vi "MatchInterface.vi"(8 "error in (no error)":errorcluster, 10 "Interface 2":T1, 11 "Interface 1":T1) -> (0 "error out":errorcluster, 2 "Wildcard":bool, 3 "Matches":bool)   [LabVIEW 2017]
uses:
  <vilib>/WebServerConfig/Interface.ctl
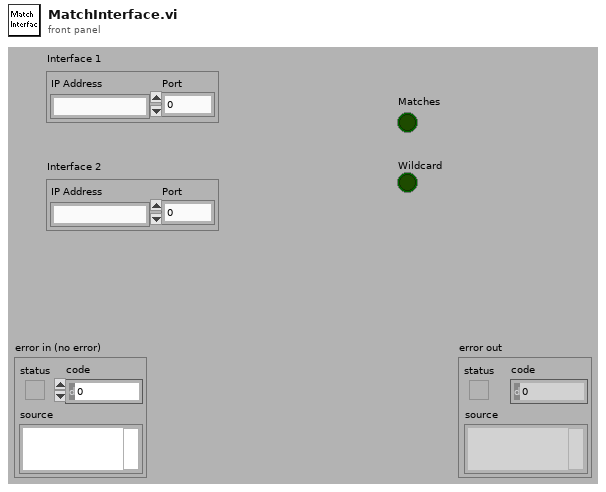
[diagram p1: front panel]
types:
  T1 = typedef "Interface.ctl" = cluster{"IP Address":string, "Port":u16}
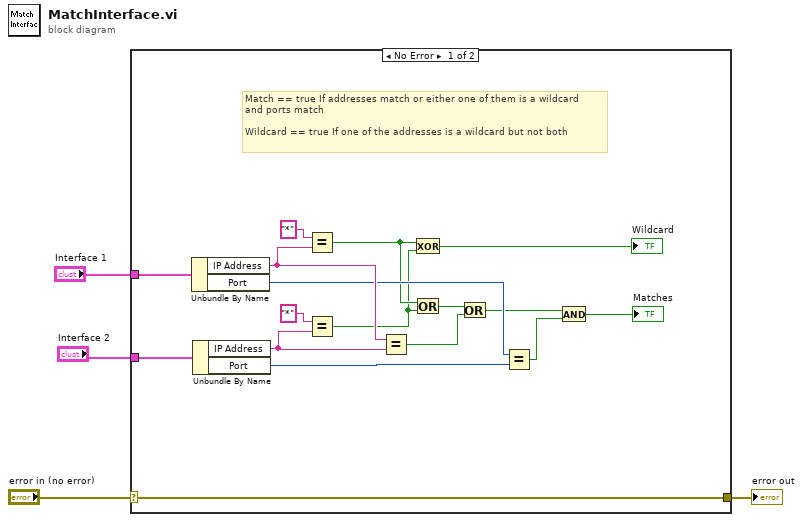
[diagram p0: block diagram]
diagram:
  n1 = case shown="No Error" "error in (no error)" {
    selector: "error in (no error)" -> [w21 w22]
    tunnel: [w21 w22] -> w3
    tunnel: "Interface 1" -> [w20 _]
    tunnel: "Interface 2" -> [w19 _]
    frame No Error {
      # "Match == true If addresses match or either one of them is a wildcard\nand ports match\n\nWildcard == true If one of the addresses is a wildcard but not both"
      n2 = Unbundle By Name(w20) -> ("IP Address"=w15:string, "Port"=w13:u16)
      n3 = Unbundle By Name(w19) -> ("IP Address"=w16:string, "Port"=w14:u16)
      n4 = Equal?(x="*", y=w15) -> (x = y?=w9:bool)
      n5 = Equal?(x="*", y=w16) -> (x = y?=w8:bool)
      n6 = Equal?(x=w15, y=w16) -> (x = y?=w11:bool)
      n7 = Exclusive Or(1:w8, 2:w9) -> (0:→"Wildcard":bool)
      n8 = Or(x=w9, y=w8) -> (x .or. y?=w6:bool)
      n9 = Or(x=w6, y=w11) -> (x .or. y?=w10:bool)
      n10 = Equal?(x=w13, y=w14) -> (x = y?=w12:bool)
      n11 = And(x=w10, y=w12) -> (x .and. y?=→"Matches":bool)
    }
    frame Error {
    }
  }
  "error out" <- w3
